vi "Number of Tests in Case.vi"() -> (3 "Number of tests":i32)   [LabVIEW 2020, in "LUnit Test Case V2 Test Double.lvclass"]
uses:
  LUnit Test Case V2 Test Double.lvclass
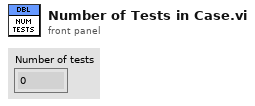
[diagram p1: front panel]
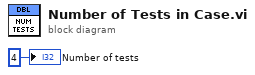
[diagram p0: block diagram]
diagram:
  "Number of tests" <- 4 ("Number of tests")
